vi "PredictedVelocityProfile (1).vi"(0 "Start Coordinate (mm)":dbl, 1 "V_Max_mm/s":dbl, 3 "Accel_mm/s^2":dbl, 5 "Target Coordinate (mm)":dbl min=0.0, 7 "error in":T1, 9 "S_Creep_mm":dbl min=0.0, 11 "S_Overrun_mm":dbl, 12 "V_Creep_mm/s":dbl, 14 "Decel_mm/s^2":dbl) -> (4 "Absolute Distance to Move (mm)":dbl, 6 "Direction Request":dbl, 8 "error out":errorcluster, 15 "PredictedVelocityProfile":cluster{dbl[], cdb[]})   [LabVIEW 2013]
uses:
  <vilib>/imath/engines/lvmath2/RunTimeEngine/ErrorHandling/NIMS_Finalize Error.vi
  <vilib>/imath/engines/lvmath2/RunTimeEngine/RangeToken/NIMS_Range.vi
  <instcachedir>/0/NIMS_Range_7481B155BEE341ECA0F59DDB444E2C09.lvgen/NIMS_Range_7481B155BEE341ECA0F59DDB444E2C09_000.vi
  <vilib>/imath/engines/lvmath2/RunTimeEngine/BuiltInFunctions/length/NIMS_length(GV).vi
  <instcachedir>/0/NIMS_length(GV)_08A3D13377FD4E4B96F5795FBF3698FA.lvgen/NIMS_length(GV)_08A3D13377FD4E4B96F5795FBF3698FA_000.vi
  <vilib>/imath/engines/lvmath2/RunTimeEngine/BuiltInFunctions/zeros/NIMS_V=zeros(I32,I32).vi
  <vilib>/imath/engines/lvmath2/RunTimeEngine/VariableToken/Support/NIMS_Vector Boolean Index to I32 Index.vi
  <vilib>/imath/engines/lvmath2/RunTimeEngine/IndexReplace/NIMS V(V)=S.vi
  <instcachedir>/0/NIMS V(V)=S_43E6004D39A2403BA86EB2871913A93B.lvgen/NIMS V(V)=S_43E6004D39A2403BA86EB2871913A93B_001.vi
  <vilib>/imath/engines/lvmath2/RunTimeEngine/ArithmeticOperatorToken/NIMS_ArithmeticOperator_power(S).vi
  <instcachedir>/0/NIMS_ArithmeticOperator_power(S)_7602F12E697C47D8910FAD43BB85D848.lvgen/NIMS_ArithmeticOperator_power(S)_7602F12E697C47D8910FAD43BB85D848_011.vi
  <vilib>/imath/engines/lvmath2/RunTimeEngine/NodeEndStatement/NIMS_NodeEndStatement_Output.vi
  <instcachedir>/0/NIMS_NodeEndStatement_Output_53EC0D466D134D7ABD903AC30B43404B.lvgen/NIMS_NodeEndStatement_Output_53EC0D466D134D7ABD903AC30B43404B_005.vi
  <instcachedir>/0/NIMS_NodeEndStatement_Output_53EC0D466D134D7ABD903AC30B43404B.lvgen/NIMS_NodeEndStatement_Output_53EC0D466D134D7ABD903AC30B43404B_000.vi
  <vilib>/imathl/engines/lvmath/Functions/Error Handling/Create Error.vi
  <instcachedir>/0/NIMS_length(GV)_08A3D13377FD4E4B96F5795FBF3698FA.lvgen/NIMS_length(GV)_08A3D13377FD4E4B96F5795FBF3698FA_002.vi
  <vilib>/imath/engines/lvmath2/RunTimeEngine/RangeToken/NIMS_Range_R2 - Integer.vi
  <instcachedir>/0/NIMS_Range_R2 - Integer_C51C130E5EA5464EA148B28CDAB9615A.lvgen/NIMS_Range_R2 - Integer_C51C130E5EA5464EA148B28CDAB9615A_000.vi
  <vilib>/imath/engines/lvmath2/RunTimeEngine/CommandStatement/MC_CommandStatement_break.vi
  <vilib>/imath/engines/lvmath2/RunTimeEngine/IndexRead/NIMS V(S).vi
  <instcachedir>/0/NIMS V(S)_0488751826AF41519A22953C041130DC.lvgen/NIMS V(S)_0488751826AF41519A22953C041130DC_003.vi
  <instcachedir>/0/NIMS_ArithmeticOperator_power(S)_7602F12E697C47D8910FAD43BB85D848.lvgen/NIMS_ArithmeticOperator_power(S)_7602F12E697C47D8910FAD43BB85D848_010.vi
  <vilib>/imath/engines/lvmath2/RunTimeEngine/IndexReplace/NIMS V(S)=S.vi
  <instcachedir>/0/NIMS V(S)=S_66A18068148B4981A312229A93EA5C06.lvgen/NIMS V(S)=S_66A18068148B4981A312229A93EA5C06_001.vi
  <vilib>/imath/engines/lvmath2/RunTimeEngine/ErrorHandling/NIMS_Create Error From Enums.vi
  <instcachedir>/0/NIMS_length(GV)_08A3D13377FD4E4B96F5795FBF3698FA.lvgen/NIMS_length(GV)_08A3D13377FD4E4B96F5795FBF3698FA_001.vi
  <instcachedir>/0/NIMS V(S)_0488751826AF41519A22953C041130DC.lvgen/NIMS V(S)_0488751826AF41519A22953C041130DC_000.vi
panel:
  out "Velocity Profile":T2(graph)
  # "Not finished, needs limits adding to inputs"
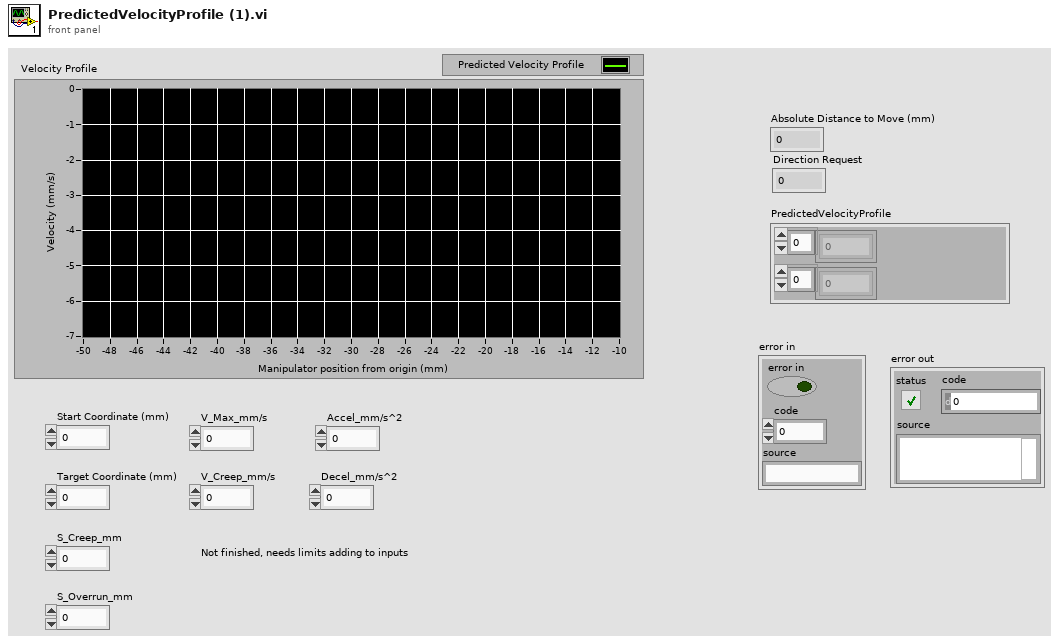
[diagram p1: front panel]
types:
  T1 = cluster{"error in":bool, "code":i32, "source":string}
  T2 = cluster{"S_DistanceArray_mm":dbl[], "V_VelocityArray_mmpers":dbl[]}
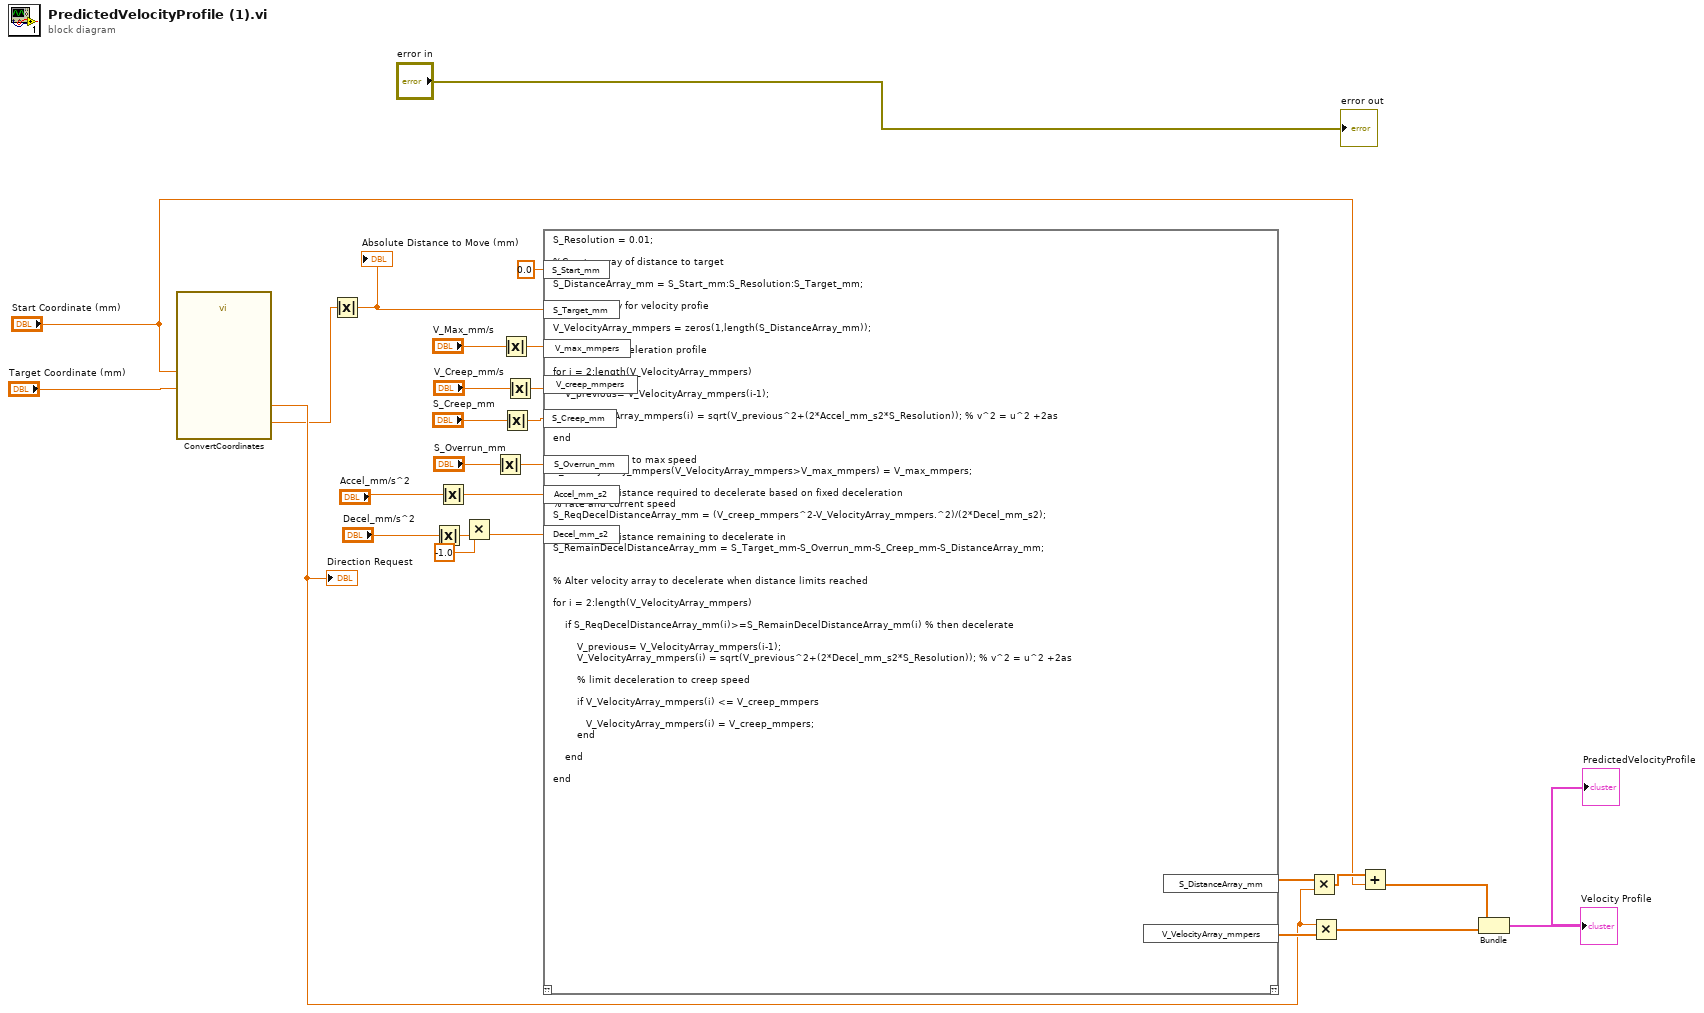
[diagram p0: block diagram]
diagram:
  n1 = call "ConvertCoordinates.vi"("Target Coordinate (mm)"="Target Coordinate (mm)", "Start Coordinate (mm)"="Start Coordinate (mm)") -> ("Direction"=w13:dbl, "Distance To Move (mm)"=w3:dbl)
  "Direction Request" <- w13
  n2 = Absolute Value(x=w3) -> (abs(x)=w2:dbl)
  "Absolute Distance to Move (mm)" <- w2
  n3 = Absolute Value(x="Decel_mm/s^2") -> (abs(x)=w10:dbl)
  n4 = Absolute Value(x="Accel_mm/s^2") -> (abs(x)=w11:dbl)
  n5 = Multiply(x=-1.0, y=w10) -> (x*y=w9:dbl)
  n6 = Absolute Value(x="S_Overrun_mm") -> (abs(x)=w4:dbl)
  n7 = Absolute Value(x="V_Max_mm/s") -> (abs(x)=w7:dbl)
  n8 = Absolute Value(x="S_Creep_mm") -> (abs(x)=w5:dbl)
  n9 = Absolute Value(x="V_Creep_mm/s") -> (abs(x)=w6:dbl)
  n10 = mathscript code="S_Resolution = 0.01;\n\n%Create array of distance to target\n\nS_DistanceArray_mm = S_Start_mm:S_Resolution:S_Target_mm;\n\n%Create array for velocity profie\n\nV_VelocityArray_mmpers = zeros(1,length(S_DistanceArray_mm));\n\n% Calculate acceleration profile\n\nfor i = 2:length(V_VelocityArray_mmpers)\n    \n    V_previous= V_VelocityArray_mmpers(i-1);\n    \n    V_VelocityArray_mmpers(i) = sqrt(V_previous^2+(2*Accel_mm_s2*S_Resolution)); % v^2 = u^2 +2as\n    \nend\n\n% Limit velocity to max speed\nV_VelocityArray_mmpers(V_VelocityArray_mmpers>V_max_mmpers) = V_max_mmpers;\n\n% Calculate distance required to decelerate based on fixed deceleration\n% rate and current speed\nS_ReqDecelDistanceArray_mm = (V_creep_mmpers^2-V_VelocityArray_mmpers.^2)/(2*Decel_mm_s2);\n\n% Calculate distance remaining to decelerate in\nS_RemainDecelDistanceArray_mm = S_Target_mm-S_Overrun_mm-S_Creep_mm-S_DistanceArray_mm;\n\n\n% Alter velocity array to decelerate when distance limits reached\n\nfor i = 2:length(V_VelocityArray_mmpers)\n    \n    if S_ReqDecelDistanceArray_mm(i)>=S_RemainDecelDistanceArray_mm(i) % then decelerate\n    \n        V_previous= V_VelocityArray_mmpers(i-1);\n        V_VelocityArray_mmpers(i) = sqrt(V_previous^2+(2*Decel_mm_s2*S_Resolution)); % v^2 = u^2 +2as\n        \n        % limit deceleration to creep speed\n        \n        if V_VelocityArray_mmpers(i) <= V_creep_mmpers\n            \n           V_VelocityArray_mmpers(i) = V_creep_mmpers;\n        end\n\n    end \n       \nend"("S_Start_mm"=0.0, "S_Target_mm"=w2, "V_max_mmpers"=w7, "V_creep_mmpers"=w6, "S_Creep_mm"=w5, "S_Overrun_mm"=w4, "Accel_mm_s2"=w11, "Decel_mm_s2"=w9) -> ("V_VelocityArray_mmpers"=w20:cdb[], "S_DistanceArray_mm"=w19:dbl[])  [unwired: 1 in, 1 out]
  n11 = Multiply(x=w19, y=w13) -> (x*y=w16:dbl[])
  n12 = Multiply(x=w13, y=w20) -> (x*y=w18:cdb[])
  n13 = Add(x=w16, y="Start Coordinate (mm)") -> (x+y=w17:dbl[])
  n14 = Bundle(w17, w18) -> (→"Velocity Profile" →"PredictedVelocityProfile":cluster{dbl[], cdb[]})  [unwired: 1 in]
  "error out" <- "error in"
